vi "AppendRunInfoH5.vi"(6 "RunInfo(clusterofbytestrings)":T1={"run_number"=1305, "LED_freq_Hz"=0.5, "LED_pulse_width_ns"=25.0, "multiplicity_requirement"=4, "HV_status"=FALSE, "start_time_UNIX"=0.0, "bytestrings"={"file_path"=[], "run_type"=[], "comments"=[], "material_in_tank"=[], "start_time_string"=[]}}, 8 "error in (no error)":errorcluster, 9 "RunInfo(strings)":T3={"run_number"=1305, "file_path"="", "LED_freq_Hz"=0.5, "LED_pulse_width_ns"=25.0, "multiplicity_requirement"=4, "HV_status"=FALSE, "run_type"="Physics", "comments"="LED width = 25 ns\n", "material_in_tank"="Water", "start_time_UNIX"=0.0, "start_time_string"=""}, 10 "RunInfo(bytestrings)":T2={"run_number"=1305, "LED_freq_Hz"=0.5, "LED_pulse_width_ns"=25.0, "multiplicity_requirement"=4, "HV_status"=FALSE, "start_time_UNIX"=0.0, "file_path"=[], "run_type"=[], "comments"=[], "material_in_tank"=[], "start_time_string"=[]}, 11 "dset in":T4 format="%.0x") -> (0 "error out":errorcluster)   [LabVIEW 2014]
uses:
  <vilib>/addons/h5labview2/base/hid_t.ctl
  <vilib>/addons/h5labview2/base/lib_path.vi
  <vilib>/addons/h5labview2/base/H5Equery.vi
  <vilib>/addons/h5labview2/dataset/H5Dwrite.llb/H5Dwrite.xnode
  <vilib>/addons/h5labview2/dataset/H5D.lvlib
  <vilib>/addons/h5labview2/space/H5S.lvlib
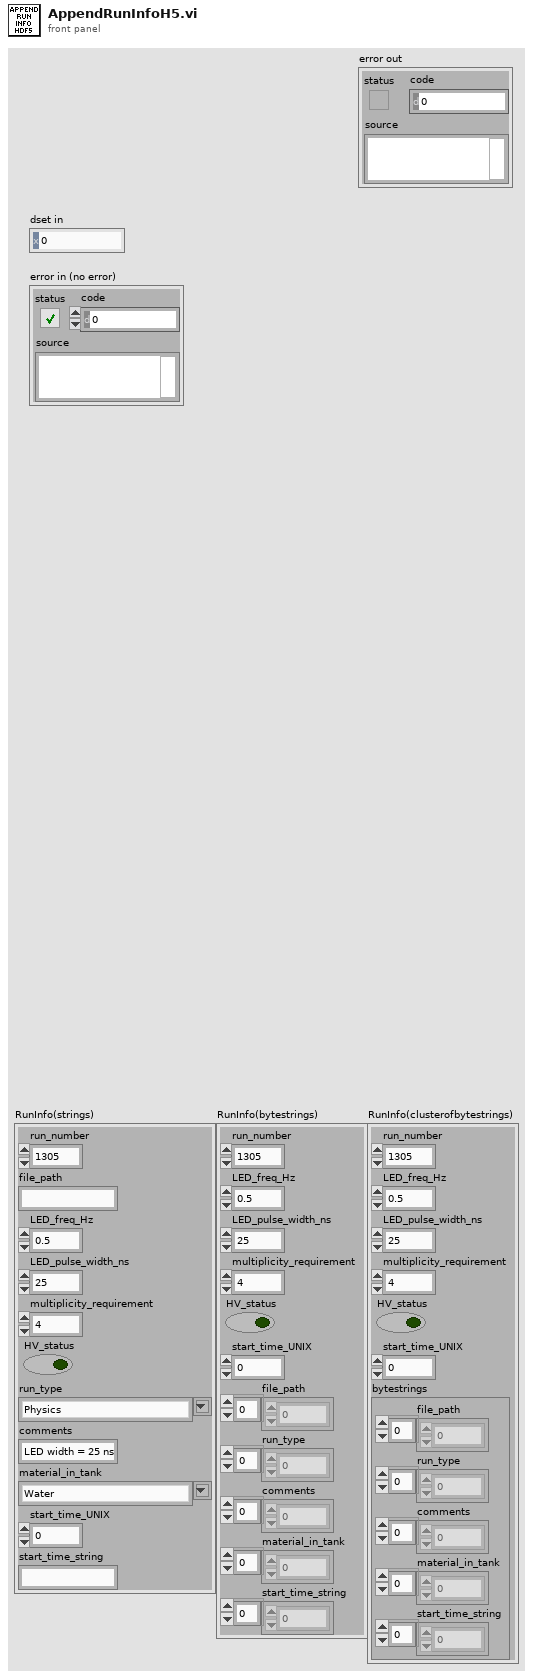
[diagram p1: front panel]
types:
  T1 = cluster{"run_number":i32, "LED_freq_Hz":dbl, "LED_pulse_width_ns":dbl, "multiplicity_requirement":u8, "HV_status":bool, "start_time_UNIX":dbl, "bytestrings":cluster{"file_path":u8[], "run_type":u8[], "comments":u8[], "material_in_tank":u8[], "start_time_string":u8[]}}
  T2 = cluster{"run_number":i32, "LED_freq_Hz":dbl, "LED_pulse_width_ns":dbl, "multiplicity_requirement":u8, "HV_status":bool, "start_time_UNIX":dbl, "file_path":u8[], "run_type":u8[], "comments":u8[], "material_in_tank":u8[], "start_time_string":u8[]}
  T3 = cluster{"run_number":i32, "file_path":string, "LED_freq_Hz":dbl, "LED_pulse_width_ns":dbl, "multiplicity_requirement":u8, "HV_status":bool, "run_type":string, "comments":string, "material_in_tank":string, "start_time_UNIX":dbl, "start_time_string":string}
  T4 = typedef "hid_t.ctl" = i32
  T5 = cluster{"run_number":i32, "file_path":string, "LED_freq_Hz":dbl, "LED_pulse_width_ns":dbl, "multiplicity_requirement":u8, "HV_status":bool, "run_type":string, "comments":string, "material_in_tank":string, "start_time_UNIX":dbl, "start_time_string":string}[]
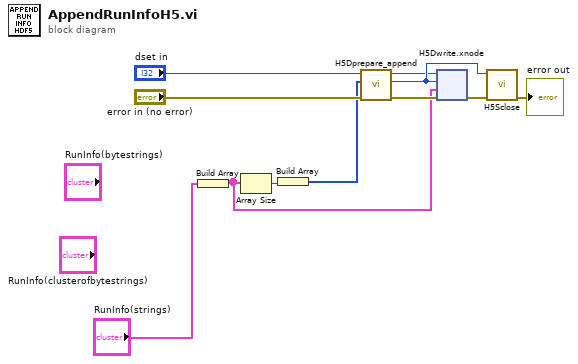
[diagram p0: block diagram]
diagram:
  n1 = Build Array("RunInfo(strings)") -> (w2:T5)
  n2 = Array Size(array=w2) -> (size(s)=w4:i32)
  n3 = Build Array(w4) -> (w3:i32[])
  n4 = call <vilib>:"H5Dprepare_append.vi"("error in (no error)"="error in (no error)", "append dims"=w3, "dset in"="dset in") -> ("error out"=w8:errorcluster, "space out"=w10:T4, "dset out"=w9:T4)  [unwired: 6 in]
  n5 = xnode "H5Dwrite.xnode"("error in (no error)"=w8, "data"=w2, "file space"=w10, "ref in"=w9) -> ("error out"=w11:errorcluster)  [unwired: 3 in, 2 out]
  n6 = call <vilib>:"H5Sclose.vi"("error in (no error)"=w11, "space in"=w10) -> ("error out"=→"error out":errorcluster)  [unwired: 9 in]
